vi "Bundle-Error.vi"(8 "error in (no error)":errorcluster, 10 "error message (\"\")":string, 11 "Errors":T1) -> (0 "error out":errorcluster)   [LabVIEW 2018, in "Scripting.lvlib"]
uses:
  Scripting.lvlib
  Error-Codes.ctl
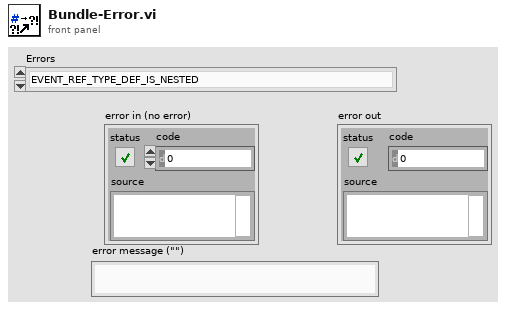
[diagram p1: front panel]
types:
  T1 = typedef "Scripting.lvlib/Error-Codes.ctl" = enum16{"EVENT_REF_TYPE_DEF_IS_NESTED", "EVENT_REF_TYPE_DEF_IS_EMPTY", "EVENT_REF_TYPE_DEF_INCLUDES_NON_REFS", "EVENT_REF_TYPE_INVALID_REPLY_REF", "EVENT_REF_TYPE_REPLY_IS_NOT_TYPE_DEF", "EVENT_REF_TYPE_DEF_IS_NOT_CLUSTER", "EVENT_REF_TYPE_DEF_INVALID_REQ_REPLY_TYPE"}
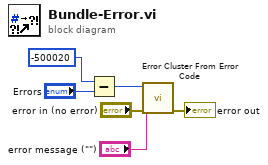
[diagram p0: block diagram]
diagram:
  n1 = Subtract(x=-500020, y="Errors") -> (x-y=w3:i32)
  n2 = call <vilib>:"Error Cluster From Error Code.vi"("error in (no error)"="error in (no error)", "error message (\"\")"="error message (\"\")", "error code (0)"=w3) -> ("error out"=→"error out":errorcluster)  [unwired: 6 in]
